vi "PumpStringAddress.vi"(11 "Pump Address":enum16{"00", "01", "02", "03"}(ring)) -> (3 "String":string)   [LabVIEW 2014]
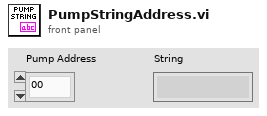
[diagram p1: front panel]
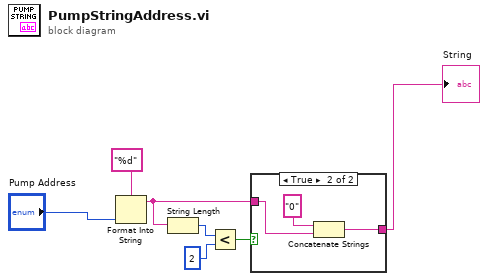
[diagram p0: block diagram]
diagram:
  n1 = Format Into String(format string="%d", "Pump Address") -> (resulting string=w5:string)  [unwired: 2 in, 1 out]
  n2 = String Length(string=w5) -> (length=w3:i32)
  n3 = Less?(x=w3, y=2) -> (x < y?=w2:bool)
  n4 = case shown="True" w2 {
    tunnel: [w8 w10] -> w7
    tunnel: w5 -> [w8 w9]
    frame False {
    }
    frame True {
      n5 = Concatenate Strings("0" ("string"), w9) -> (w10:string)
    }
  }
  "String" <- w7
